vi "Verify position.vi"(8 "error in (no error)":errorcluster, 9 "Tolerance (um)":sgl=0.4, 10 "XYZ Position Input":T2={"Speed"=0, "Z Limit (um+/-)"=0.0, "Axes"="Z", "XYZ Coordinates"={"X"=0.0, "Y"=0.0, "Z"=0.0}} {"XYZ Coordinates"."Z" format="Z= %#_g"; "XYZ Coordinates"."Y" format="Y= %#_g"; "XYZ Coordinates"."X" format="X= %#_g"; "Z Limit (um+/-)" format="Z Limit = %.0f"; "Speed" format="Speed= %.0f"}, 11 "XYZ Stage Control in":refnum<class "XYZ Stage Control.lvclass">) -> (0 "error out":errorcluster, 1 "XYZ Coordinates":T1 {"Z" format="Z= %#_g"; "Y" format="Y= %#_g"; "X" format="X= %#_g"}, 2 "Position reached":bool, 3 "XYZ Stage Control out":refnum<class "XYZ Stage Control.lvclass">)   [LabVIEW 2020, in "TranslationStageClassStructure.lvlib" / "XYZ Stage Control.lvclass"]
uses:
  XYZ Stage Control.lvclass
  typedefs/XYZ_position_input.ctl
  typedefs/XYZ axes.ctl
  Typedefs/XYZ_coordinates.ctl
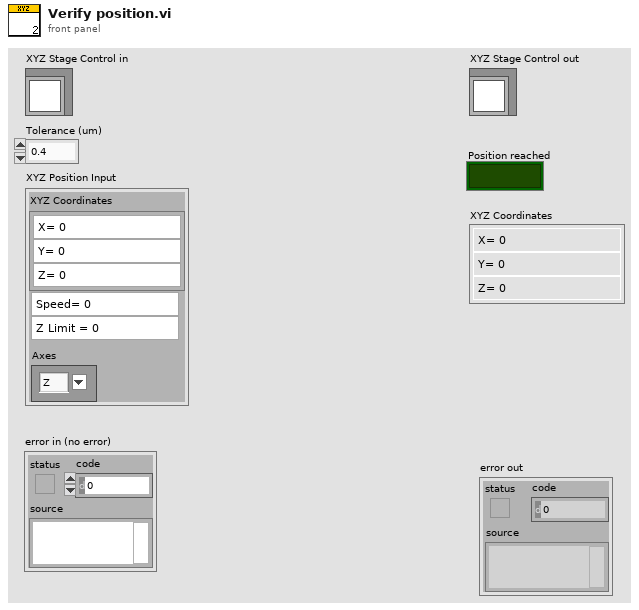
[diagram p1: front panel]
types:
  T1 = typedef "XYZ_coordinates.ctl" = cluster{"X":sgl, "Y":sgl, "Z":sgl}
  T2 = typedef "XYZ_position_input.ctl" = cluster{"Speed":i32, "Z Limit (um+/-)":sgl, "Axes":T3, "XYZ Coordinates":T1}
  T3 = typedef "XYZ axes.ctl" = string
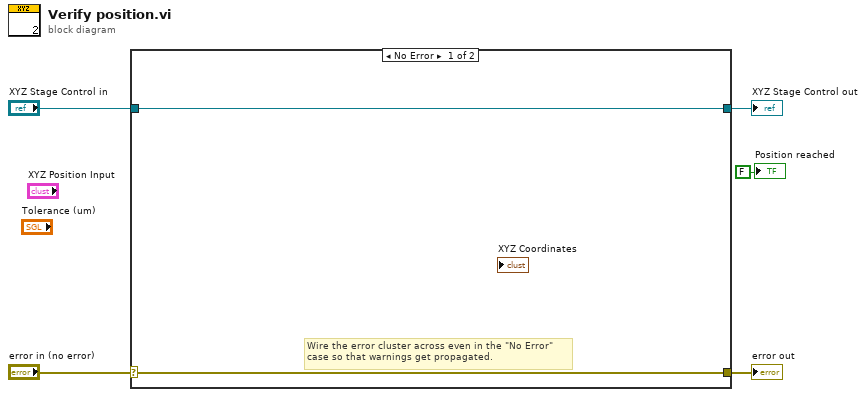
[diagram p0: block diagram]
diagram:
  n1 = case shown="No Error" "error in (no error)" {
    selector: "error in (no error)" -> [w6 w9]
    tunnel: [w6 w9] -> w4
    tunnel: [w7 w8] -> w2
    tunnel: "XYZ Stage Control in" -> [w7 w8]
    frame No Error {
      # "Wire the error cluster across even in the \"No Error\"\ncase so that warnings get propagated."
    }
    frame Error {
    }
  }
  "error out" <- w4
  "XYZ Stage Control out" <- w2
  "Position reached" <- FALSE ("Position reached")
